vi "Task Loop.vi"(8 "error in (no error)":errorcluster, 11 "DaqControl in":refnum<class "DaqControl.lvclass">) -> (0 "error out":errorcluster)   [LabVIEW 2020, in "VolatusDaq.lvlib" / "DaqControl.lvclass"]
uses:
  DaqControl.lvclass
  <vilib>/Platform/TimedLoop/XDataNode/timing_clust.ctl
  <vilib>/Platform/TimedLoop/XDataNode/nitl_modes.ctl
  <vilib>/Platform/TimedLoop/XDataNode/wakeup.ctl
  Volatus/DataHandlerAPI/DataHandlerAPI.lvclass/DataHandlerAPI.ctl
  Volatus/DataHandler Messages/New Data Msg/New Data Msg.lvclass/New Data Msg.ctl
  <vilib>/ActorFramework/Message Enqueuer/Message Enqueuer.lvclass/Message Enqueuer.ctl
  Volatus/Event API/EventAPI.lvclass/EventAPI.ctl
  Volatus/EventHandler Messages/Handle Event Msg/Handle Event Msg.lvclass/Handle Event Msg.ctl
  <vilib>/DAQmx/write.llb/DAQmx Write.vi
  <vilib>/DAQmx/write.llb/DAQmx Write (Analog 1D DBL NChan 1Samp).vi
  <vilib>/DAQmx/write.llb/DAQmx Write (Digital 1D Bool NChan 1Samp 1Line).vi
  Control Loop Status Values.vi
  Volatus/Event API/Report Error.vi
  Volatus/DataHandlerAPI/New Data.vi
  lv-vecto/Vecto/Bool to Double.vi
  Volatus/Event API/Report Event.vi
  Volatus/DataHandler Messages/New Data Msg/Send New Data.vi
  Volatus/EventHandler Messages/Handle Event Msg/Send Handle Event.vi
  <vilib>/ActorFramework/Message Enqueuer/Enqueue.vi
  Volatus/DataHandler Messages/New Data Msg/New Data Msg.lvclass
  C:/Program Files (x86)/National Instruments/LabVIEW 2020/vi.lib/ActorFramework/Message/Message.lvclass
  Volatus/EventHandler Messages/Handle Event Msg/Handle Event Msg.lvclass
  <vilib>/DAQmx/miscellaneous.llb/DAQmx Fill In Error Info.vi
  <vilib>/ActorFramework/Message Priority Queue/Priority Enqueue.vi
  <vilib>/platform/TimedLoop/XDataNode/XDataNode.xnode
  DaqControl.lvclass/DaqControl.ctl
  <vilib>/Platform/TimedLoop/XDataNode/XDNodeRunTimeDep.lvlib
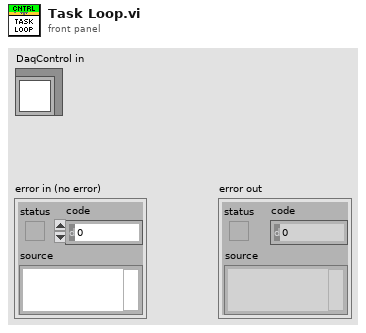
[diagram p1: front panel]
types:
  T1 = typedef "XDNodeRunTimeDep.lvlib/timing_clust.ctl" = cluster{"Expected End [f-1]":u64, "Actual End [f-1]":u64, "Finished Late? [f-1]":bool, "Expected End [i-1]":u64, "Actual End [i-1]":u64, "Finished Late? [i-1]":bool, "Expected Start [i]":u64, "Actual Start [i]":u64, "Expected Start [f]":u64, "Actual Start [f]":u64, "Source Name":string, "Structure Name":string, "Period":i64, "Deadline":i64, "Offset":i64, "Start":i64, "Priority":i32, "Timeout":i32, "Mode":T2, "Wakeup Reason":T3, "Error":errorcluster, "Source Type":string, "Secondary Source Type":string, "Global End Time":u64, "Global Start Time":u64, "Frame Duration":u64, "Iteration Duration":u64, "Assigned CPU":i32, "I/O Scan Engine Mode":u32}
  T2 = typedef "XDNodeRunTimeDep.lvlib/nitl_modes.ctl" = enum32{"No Change", "Process missed periods, maintain original phase", "Discard missed periods, maintain original phase", "Process missed periods, ignore original phase", "Discard missed periods, ignore original phase"}
  T3 = typedef "XDNodeRunTimeDep.lvlib/wakeup.ctl" = enum32{"Normal", "Aborted", "Asynchronous wakeup", "Timing source error", "Timed loop error", "Timeout"}
  T4 = typedef "VolatusDaq.lvlib/DaqControl.lvclass/Loop Data.ctl" = cluster{"Values":dbl[], "Ticks":u32, "Auto":bool, "Ticks Start":u32, "Abort":bool, "Value Cmd Q":refnum<queue>, "Seq Index":i32, "Seq Cmd Q":refnum<queue>, "DAQmx":refnum<k21>, "Signal Type":T5, "EventAPI":refnum<class "EventAPI.lvclass">, "Name":string, "Stop Notifier":refnum<notifier>, "Logger":refnum<class "DataHandlerAPI.lvclass">, "Sequence":T6}
  T5 = typedef "VolatusDaq.lvlib/Signal Type.ctl" = enum16{"Analog", "Digital"}
  T6 = typedef "VolatusDaq.lvlib/Sequence.ctl" = cluster{"Run":T7[], "Abort":T7[]}
  T7 = typedef "VolatusDaq.lvlib/Sequence Action.ctl" = cluster{"Tick":u32, "Seq Action Type":T8, "Index Param":i32, "Value Param":dbl}
  T8 = typedef "VolatusDaq.lvlib/Seq Action Type.ctl" = enum16{"Value", "Stop"}
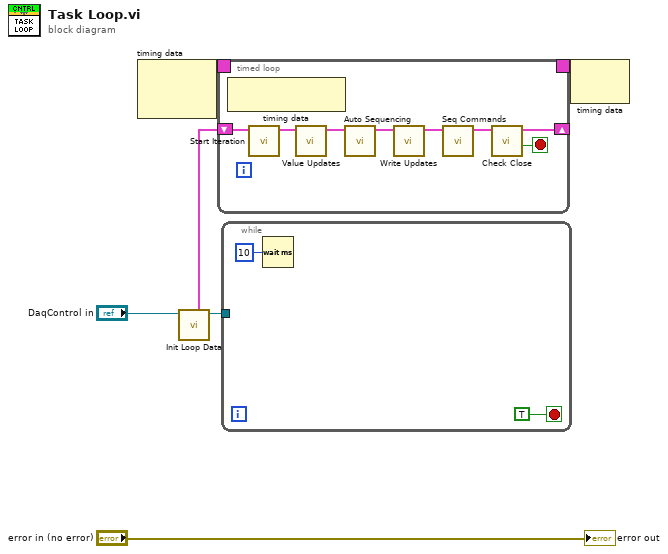
[diagram p0: block diagram]
diagram:
  n1 = node-c288() -> (w6:T1)  [unwired: 2 in]
  n2 = call "Init Loop Data.vi"("DaqControl in"="DaqControl in") -> ("DaqControl out"=w1:refnum<class "DaqControl.lvclass">, "Loop Data"=w2:T4)  [unwired: 8 in, 1 out]
  n3 = timed-loop {
    timing: w6 -> [_]
    timing-out: [_] -> w5
    shift-right: [w8] -> _
    shift-left: w2 -> [w13]
    stop <- w7 stop-if-true
    n4 = node-c288() -> ()  [unwired: 1 in, 1 out]
    n5 = call "Start Iteration.vi"("Loop Data in"=w13) -> ("Loop Data"=w10:T4)  [unwired: 10 in]
    n6 = call "Value Updates.vi"("DaqControl in"=w10) -> ("DaqControl out"=w14:T4)  [unwired: 10 in]
    n7 = call "Auto Sequencing.vi"("DaqControl in"=w14) -> ("DaqControl out"=w12:T4)  [unwired: 10 in]
    n8 = call "Write Updates.vi"("DaqControl in"=w12) -> ("DaqControl out"=w11:T4)  [unwired: 10 in]
    n9 = call "Seq Commands.vi"("Loop Data in"=w11) -> ("Loop Data"=w9:T4)  [unwired: 10 in]
    n10 = call "Check Close.vi"("DaqControl in"=w9) -> ("Stop"=w7:bool, "DaqControl out"=w8:T4)  [unwired: 9 in]
  }
  n11 = while {
    tunnel: w1 -> [_]
    stop <- TRUE stop-if-true
    n12 = Wait (ms)(milliseconds to wait=u32 10) -> ()  [unwired: 1 out]
  }
  n13 = node-c288(w5) -> ()  [unwired: 1 out]
  "error out" <- "error in (no error)"
